vi "Ethernet IP Global Tag Array.vi"() -> ()   [LabVIEW 2011, in "Ethernet IP Custom Device Custom Device.lvlib"]
uses:
  Ethernet IP Custom Device Custom Device.lvlib
  L5K Internal Data.ctl
  L5K Tag.ctl
  L5K Data Types.ctl
panel:
  in  "Tags not imported":string
  out "L5K Information":T1
  in  "Tag Info for MCLB":string[][](array[string])=[["", "Tag_BOOL", "BOOL", "1"], ["", "Tag_BOOL_Array", "BOOL", "32"], ["", "Tag_BOOL_ArrayLong", "BOOL", "96"], ["", "Tag_BOOL_ShortArray", "BOOL", "32"], ["", "Tag_BOOL_Unconnected", "BOOL", "1"], ["", "Tag_DINT", "DINT", "1"], ["", "Tag_DINT_Array", "DINT", "3"], ["", "Tag_INT", "INT", "1"], ["", "Tag_INT_Array", "INT", "3"], ["", "Tag_REAL", "REAL", "1"], ["", "Tag_REAL_Array", "REAL", "3"], ["", "Tag_SINT", "SINT", "1"], ["", "Tag_SINT_Array", "SINT", "3"], ["", "Tag_STRING", "STRING", "1"], ["", "Tag_STRING_Array", "STRING", "1"]]
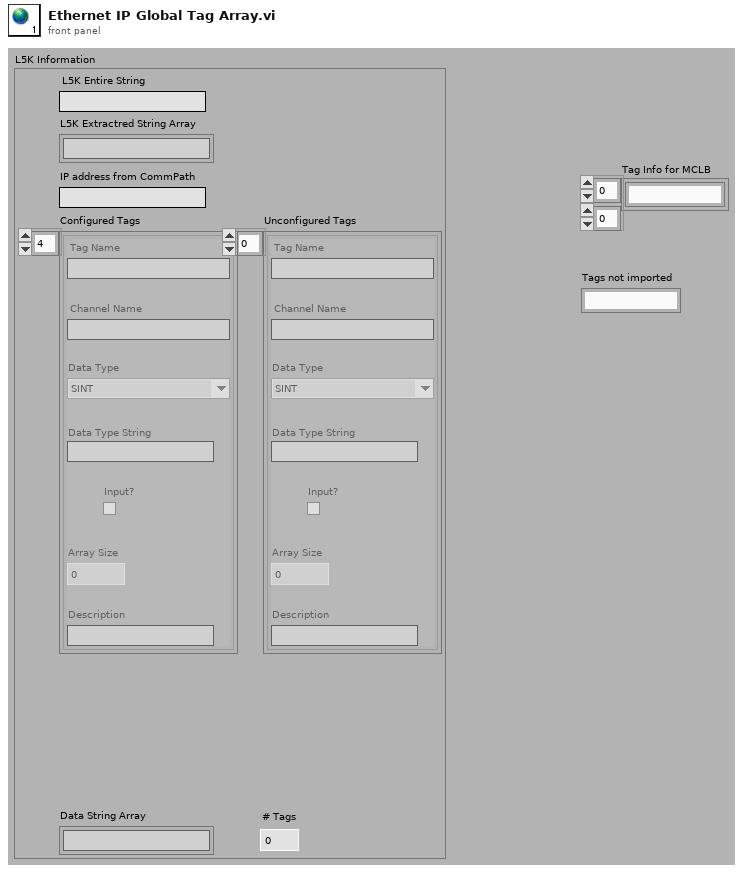
[diagram p1: front panel]
types:
  T1 = typedef "Ethernet IP Custom Device Custom Device.lvlib/L5K Internal Data.ctl" = cluster{"L5K Entire String":string, "L5K Extractred String Array":string[], "IP address from CommPath":string, "Configured Tags":T2[], "Data String Array":string[], "Unconfigured Tags":T2[], "# Tags":i32}
  T2 = typedef "Ethernet IP Custom Device Custom Device.lvlib/L5K Tag.ctl" = cluster{"Tag Name":string, "Data Type":T3, "Data Type String":string, "Array Size":i32, "Description":string, "Input?":bool, "Channel Name":string}
  T3 = typedef "Ethernet IP Custom Device Custom Device.lvlib/L5K Data Types.ctl" = enum16{"SINT", "INT", "DINT", "REAL", "BOOL"}
diagram:
